vi "Create.vi"(7 "options":T1={"FIFO Options"={"Infinite Timeouts"=FALSE}, "Thread Options"={"Show FP On Call"=FALSE, "Close FP After Call"=FALSE, "Allow Debugging"=FALSE}, "Plugin Options"={"Default Components"=FALSE}, "Performance Options"={"Measure Period"=FALSE, "Measure Rx/Tx Duration"=FALSE}, "Data Server Options"={"Enable Data Server"=FALSE, "Period"=50}} {"Data Server Options"."Period" format="%d ms"}, 8 "error in (no error)":errorcluster, 11 "Device Item Ref":T7=18446744073709551615 format="%.0x") -> (0 "error out":errorcluster, 3 "VeriStand Framework":refnum<class "VeriStand DSF.lvclass">)   [LabVIEW 2020, in "DSF Engine.lvlib" / "VeriStand DSF.lvclass"]
uses:
  VeriStand DSF.lvclass
  <vilib>/NI VeriStand/Custom Device API/Custom Device Item Ref.ctl
  Includes/DSF Core.lvlibp/Classes/Framework/Framework Options.ctl
  Includes/DSF Core.lvlibp/Typedefs/DSF FIFO Options.ctl
  Includes/DSF Core.lvlibp/Classes/Thread/Thread Options.ctl
  Includes/DSF Core.lvlibp/Typedefs/DSF Plugin Options.ctl
  Includes/DSF Core.lvlibp/Typedefs/DSF Performance Options.ctl
  Includes/DSF Core.lvlibp/Classes/Framework/Data Server Options.ctl
  VeriStand DSF.lvclass/VeriStand DSF.ctl
  Shared/DSF Shared.lvlib
  Includes/DSF Core.lvlibp/Classes/Configuration/Core/Framework/Framework Configuration.lvclass
  <vilib>/NI VeriStand/Custom Device API/Custom Device API.lvlib
  Includes/DSF Core.lvlibp/Classes/Framework/Framework.lvclass
  Includes/DSF Core.lvlibp
  Includes/DSF Core.lvlibp/Classes/Thread/Thread.lvclass
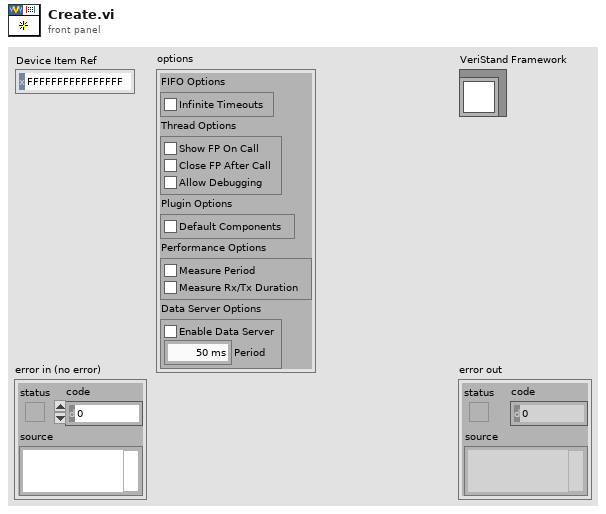
[diagram p1: front panel]
types:
  T1 = typedef "DSF Core.lvlibp/Framework.lvclass/Framework Options.ctl" = cluster{"FIFO Options":T2, "Thread Options":T3, "Plugin Options":T4, "Performance Options":T5, "Data Server Options":T6}
  T2 = typedef "DSF Core.lvlibp/Framework.lvclass/DSF FIFO Options.ctl" = cluster{"Infinite Timeouts":bool}
  T3 = typedef "DSF Core.lvlibp/Thread.lvclass/Thread Options.ctl" = cluster{"Show FP On Call":bool, "Close FP After Call":bool, "Allow Debugging":bool}
  T4 = typedef "DSF Core.lvlibp/Framework.lvclass/DSF Plugin Options.ctl" = cluster{"Default Components":bool}
  T5 = typedef "DSF Core.lvlibp/DSF Performance Options.ctl" = cluster{"Measure Period":bool, "Measure Rx/Tx Duration":bool}
  T6 = typedef "DSF Core.lvlibp/Framework.lvclass/Data Server Options.ctl" = cluster{"Enable Data Server":bool, "Period":u32}
  T7 = typedef "Custom Device API.lvlib/Custom Device Item Ref.ctl" = u64
  T8 = typedef "DSF Core.lvlibp/DSF Engine Framework Configuration.ctl" = cluster{"plugins":T9[]}
  T9 = typedef "DSF Core.lvlibp/DSF Engine Plugin Configuration.ctl" = cluster{"core":T10, "component settings":T12[], "threads":T13[]}
  T10 = typedef "DSF Core.lvlibp/Plugin Configuration.lvclass/Core Plugin Configuration.ctl" = cluster{"name":string, "components":string[], "cycle timing":T11}
  T11 = typedef "DSF Core.lvlibp/DSF Timing Info.ctl" = cluster{"priority":u64, "decimation":u64, "offset":u64}
  T12 = typedef "DSF Core.lvlibp/DSF Settings Info.ctl" = cluster{"component":string, "values":cluster{"key":string, "value":string}[]}
  T13 = typedef "DSF Core.lvlibp/DSF Engine Plugin Thread Configuration.ctl" = cluster{"core":T14, "component settings":T12[], "transfer groups":T15[]}
  T14 = typedef "DSF Core.lvlibp/Thread Configuration.lvclass/Core Thread Configuration.ctl" = cluster{"processor":i32, "priority offset":i16}
  T15 = typedef "DSF Core.lvlibp/DSF Engine Transfer Group Configuration.ctl" = cluster{"core":T16, "component settings":T12[], "transfers":T19[]}
  T16 = typedef "DSF Core.lvlibp/Group Configuration.lvclass/Core Group Configuration.ctl" = cluster{"name":string, "direction":T17, "cycle timing":T11, "timeout behavior":T18, "enable conversion":bool}
  T17 = typedef "DSF Core.lvlibp/DSF Direction.ctl" = enum8{"Tx", "Rx"}
  T18 = typedef "DSF Core.lvlibp/DSF Timeout Behavior.ctl" = enum8{"Increment Late Count", "Throw Error"}
  T19 = typedef "DSF Core.lvlibp/DSF Engine Transfer Configuration.ctl" = cluster{"core":T20, "component settings":T12[], "channels":T21[]}
  T20 = typedef "DSF Core.lvlibp/Transfer Configuration.lvclass/Core Transfer Configuration.ctl" = cluster{"name":string}
  T21 = typedef "DSF Core.lvlibp/DSF Engine Channel Configuration.ctl" = cluster{"core":T22, "component settings":T12[]}
  T22 = typedef "DSF Core.lvlibp/Channel Configuration.lvclass/Core Channel Configuration.ctl" = cluster{"name":string, "units":string, "engine data type":T23, "string data type":T23, "string offset":u64}
  T23 = typedef "DSF Core.lvlibp/DSF Data Type.ctl" = enum8{"Bool", "SGL", "DBL", "I8", "I16", "I32", "I64", "U8", "U16", "U32", "U64"}
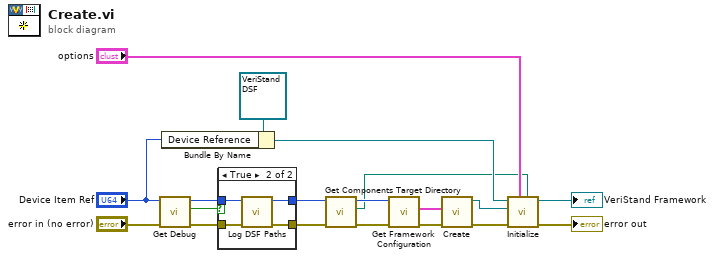
[diagram p0: block diagram]
diagram:
  n1 = call "Get Debug.vi"("error in (no error)"="error in (no error)", "Item Ref in"="Device Item Ref") -> ("error out"=w12:errorcluster, "debug"=w11:bool, "Item Ref out"=w13:T7)  [unwired: 7 in]
  n2 = Bundle By Name(cluster=refnum<class "VeriStand DSF.lvclass"> refnum ("VeriStand Data Sharing Framework out"), "Device Reference"="Device Item Ref") -> (w18:refnum<class "VeriStand DSF.lvclass">)
  n3 = case shown="True" w11 {
    tunnel: w13 -> [w21 w25]
    tunnel: w12 -> [w20 w24]
    tunnel: [w21 w23] -> w9
    tunnel: [w20 w22] -> w10
    frame False {
    }
    frame True {
      n4 = call "Log DSF Paths.vi"("error in (no error)"=w24, "Item Ref in"=w25) -> ("error out"=w22:errorcluster, "Item Ref out"=w23:T7)  [unwired: 8 in]
    }
  }
  n5 = call "Get Components Target Directory.vi"("error in (no error)"=w10, "Item Ref in"=w9) -> ("error out"=w5:errorcluster, "components target directory"=w1:path, "Item Ref out"=w2:T7)  [unwired: 7 in]
  n6 = call "Get Framework Configuration.vi"("error in (no error)"=w5, "Item Ref in"=w2) -> ("error out"=w4:errorcluster, "framework configuration"=w3:T8)  [unwired: 7 in, 1 out]
  n7 = call "Create.vi"("error in (no error)"=w4, "framework configuration"=w3) -> ("error out"=w6:errorcluster, "Framework Configuration out"=w7:refnum<class "Framework Configuration.lvclass">)  [unwired: 8 in]
  n8 = call-dynamic "Initialize.vi"("components directory"=w1, "options"="options", "error in (no error)"=w6, "Framework Configuration"=w7, "VeriStand DSF in"=w18) -> ("error out"=→"error out":errorcluster, "VeriStand DSF out"=→"VeriStand Framework":refnum<class "VeriStand DSF.lvclass">)  [unwired: 5 in]
